vi "Framework_Initialize.vi"(8 "error in (no error)":errorcluster, 11 "AB_DepPackedLibrary in":refnum<class "AB_DepPackedLibrary.lvclass">) -> (0 "error out":errorcluster, 1 "helpTopics":string[](array[string]), 2 "pageTitles":string[](array[string]), 3 "AB_DepPackedLibrary out":refnum<class "AB_DepPackedLibrary.lvclass">, 4 "helpFile":string, 5 "pages":path[](array[path]))   [LabVIEW 2020, in "AB_DepPackedLibrary.lvclass"]
uses:
  <vilib>/AppBuilder/AB_Classes/DepPackedLib/AB_DepPackedLibrary.lvclass
  <vilib>/AppBuilder/AB_Classes/PackedLib/AB_PackedLibrary.lvclass
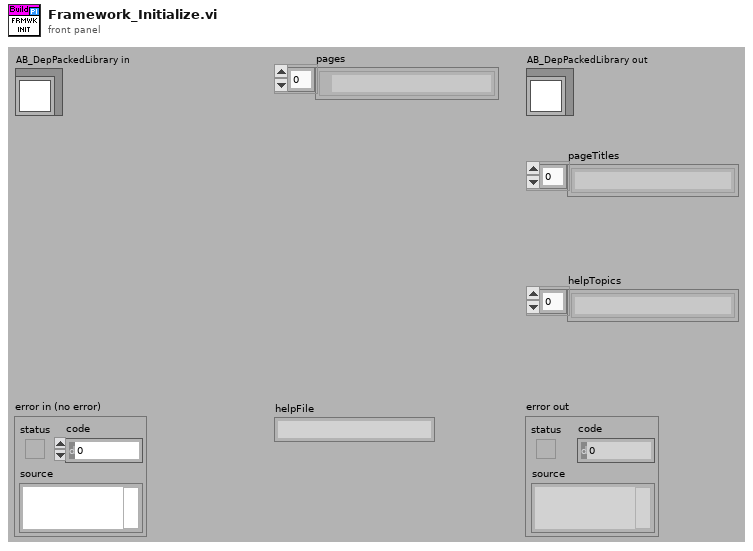
[diagram p1: front panel]
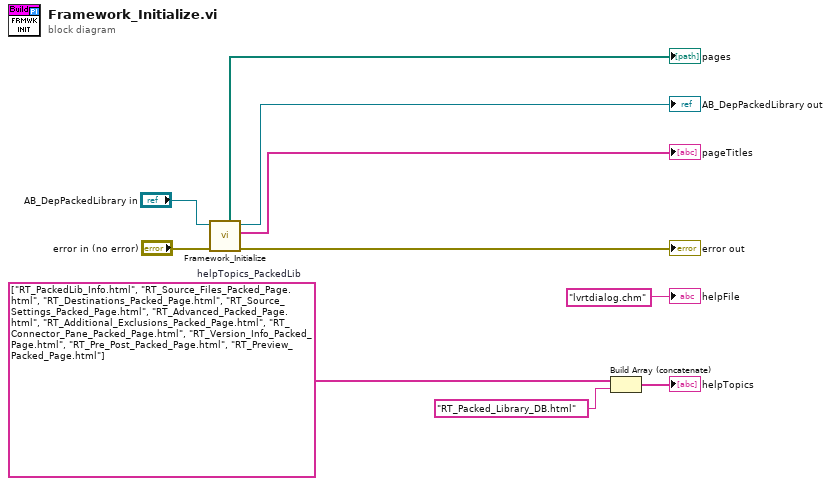
[diagram p0: block diagram]
diagram:
  w3 = string[] ["RT_PackedLib_Info.html", "RT_Source_Files_Packed_Page.html", "RT_Destinations_Packed_Page.html", "RT_Source_Settings_Packed_Page.html", "RT_Advanced_Packed_Page.html", "RT_Additional_Exclusions_Packed_Page.html", "RT_Connector_Pane_Packed_Page.html", "RT_Version_Info_Packed_Page.html", "RT_Pre_Post_Packed_Page.html", "RT_Preview_Packed_Page.html"]  # helpTopics_PackedLib
  n1 = call-parent "Framework_Initialize.vi"("error in (no error)"="error in (no error)", "AB_PackedLibrary in"="AB_DepPackedLibrary in") -> ("error out"=→"error out":errorcluster, "pageTitles"=→"pageTitles":string[], "AB_PackedLibrary out"=→"AB_DepPackedLibrary out":refnum<class "AB_DepPackedLibrary.lvclass">, "pages"=→"pages":path[])  [unwired: 4 in, 2 out]
  n2 = Build Array (concatenate)(w3, "RT_Packed_Library_DB.html" ("HTML filename")) -> (→"helpTopics":string[])
  "helpFile" <- "lvrtdialog.chm" ("CHM or HLP filename (lvdialog.chm)")
